vi "C to F.vi"(1 "DEG C":dbl) -> (0 "Deg F":dbl)   [LabVIEW 2015]
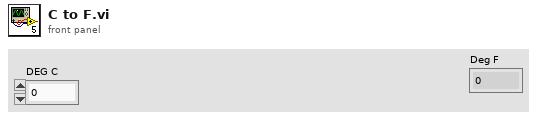
[diagram p1: front panel]
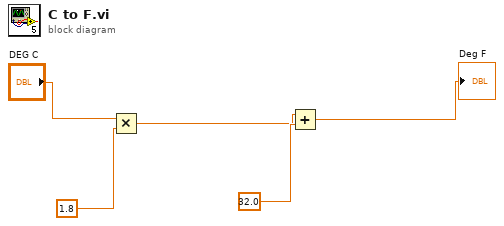
[diagram p0: block diagram]
diagram:
  n1 = Multiply(x="DEG C", y=1.8) -> (x*y=w2:dbl)
  n2 = Add(x=w2, y=32.0) -> (x+y=→"Deg F":dbl)
